vi "AIT 1553 - Check Valid License.vi"(11 "error in (no error)":errorcluster) -> (4 "activation successful?":bool, 6 "activated?":bool, 15 "error out":errorcluster)   [LabVIEW 2015, in "AIT 1553 Custom Device.lvlib"]
uses:
  AIT 1553 Custom Device.lvlib
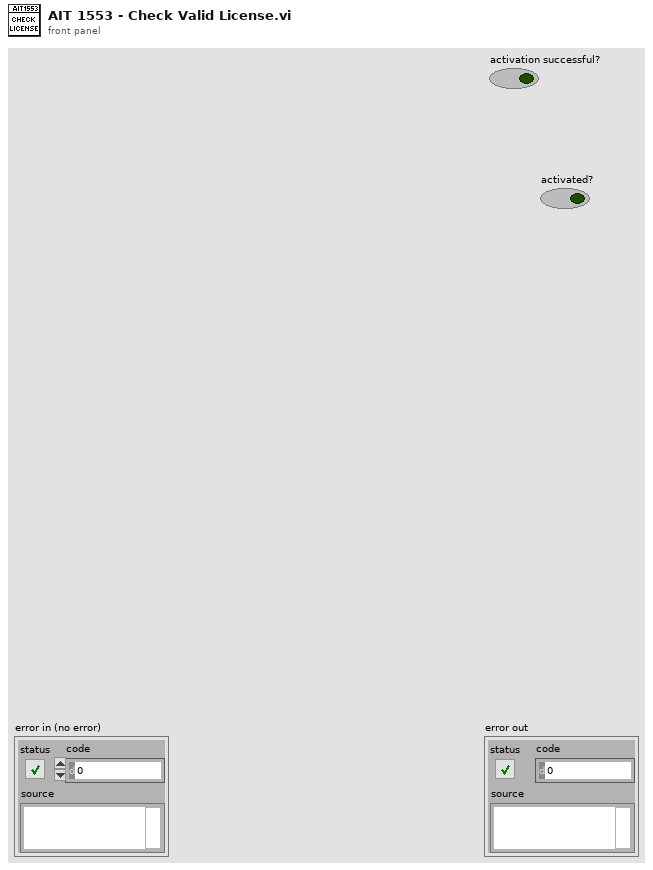
[diagram p1: front panel]
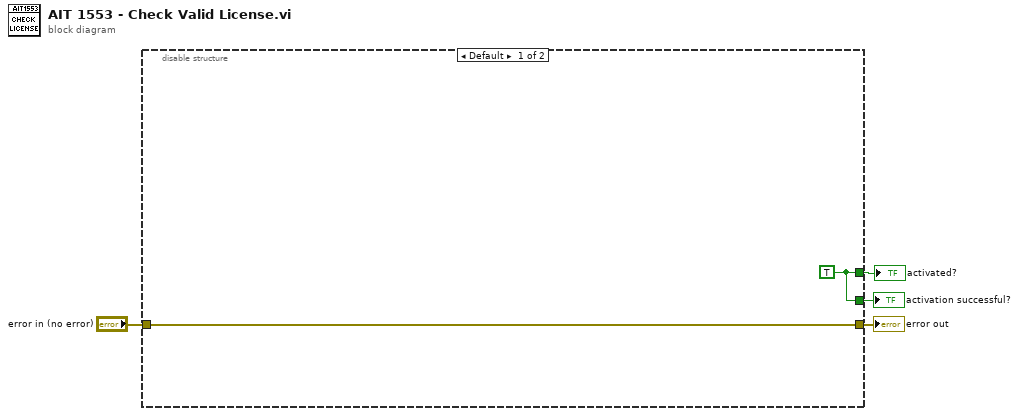
[diagram p0: block diagram]
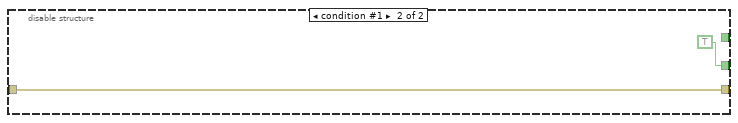
[diagram p2: hidden frame]
diagram:
  n1 = disable-structure shown="Default" {
    disable-tunnel: [w6 TRUE ("activation successful?")] -> w4
    disable-tunnel: [w5 w7] -> w3
    disable-tunnel: "error in (no error)" -> [w5 w7]
    disable-tunnel: [w6 _] -> w1
    frame condition #0 (active) {
      w6 = TRUE ("activated?")
    }
    frame condition #1 {
    }
  }
  "activation successful?" <- w4
  "error out" <- w3
  "activated?" <- w1
